vi "Get Scaling Parameters (User Defined).vi"(0 "session in":refnum<k21>, 5 "physical channel":refnum<k21>="$DefaultPhysChans", 11 "error in (no error)":errorcluster) -> (4 "session out":refnum<k21>, 6 "physical channel out":refnum<k21>, 8 "parameter names":string[](array[string]), 10 "parameter values":dbl[](array[numeric]), 15 "error out":errorcluster)   [LabVIEW 2020, in "SLSC.lvlib"]
doc: "Gets scaling parameters from a user-defined scale."
uses:
  <vilib>/SLSC/SLSC.lvlib
  nislsclvapi.dll
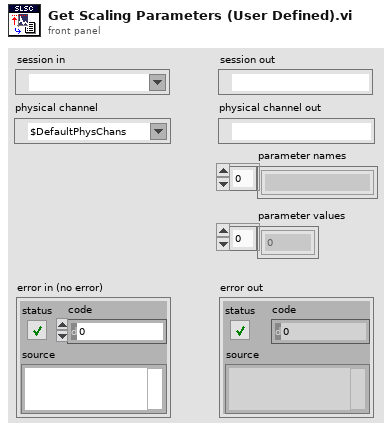
[diagram p1: front panel]
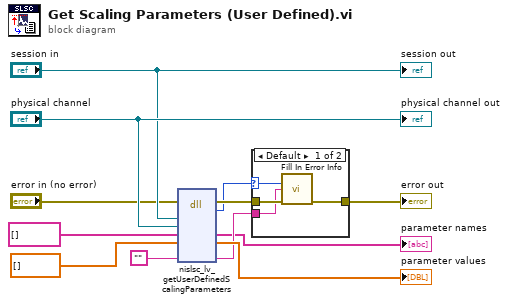
[diagram p0: block diagram]
diagram:
  n1 = dll-call lib="nislsclvapi.*" fn="nislsc_lv_getUserDefinedScalingParameters"(error in="error in (no error)", "session"="session in", "physical channel"="physical channel", "parameternames"=string[] [] ("parameter names"), "parametervalues"=dbl[] [], "extendedErrorInfo"="") -> (error out=w5:errorcluster, "return type"=w3:i32, "parameternames"=→"parameter names":string[], "parametervalues"=→"parameter values":dbl[], "extendedErrorInfo"=w4:string)  [unwired: 6 in, 1 out]
  n2 = case shown="Default" w3 {
    selector: w3 -> [w13 _]
    tunnel: w4 -> [w14 _]
    tunnel: w5 -> [w16 w17]
    tunnel: [w15 w17] -> w6
    frame Default {
      n3 = call <vilib>:"Fill In Error Info.vi"("status code"=w13, "extended error info"=w14, "error in"=w16) -> ("error out"=w15:errorcluster)  [unwired: 12 in]
    }
    frame 0 {
    }
  }
  "error out" <- w6
  "session out" <- "session in"
  "physical channel out" <- "physical channel"
